vi "Test Panel Wavelength.vi"(8 "error in (no error)":errorcluster, 11 "VISA resource name":refnum<visa-resource-name>="COM4") -> (0 "error out":errorcluster, 3 "VISA resource name out":refnum<visa-resource-name>)   [LabVIEW 2017]
panel:
  out "Wavelength":dbl[unit]
  in  "Numeric":i32
  in  "stop":bool
  out "query output":string
  out "read buffer 3":string
  in  "wavelength":dbl[unit] min=0.0 max=1.99999e-05 step=1.0000000000000002e-10
  out "Boolean":bool
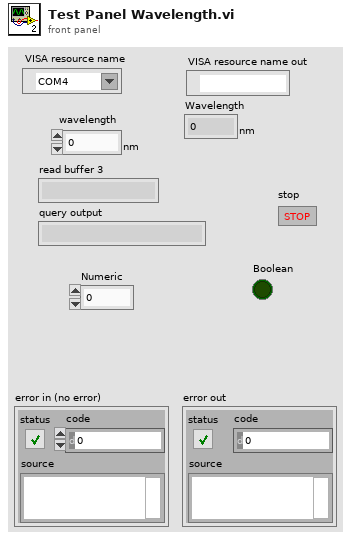
[diagram p1: front panel]
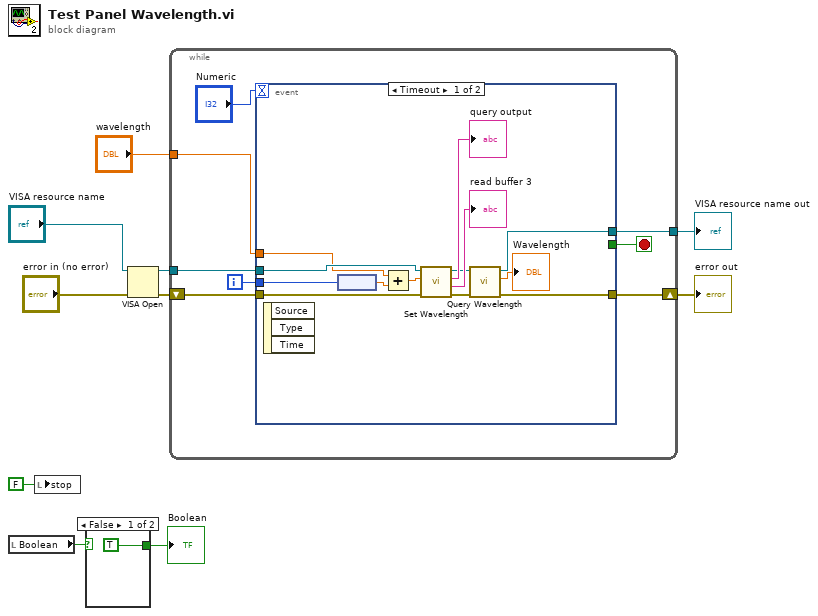
[diagram p0: block diagram]
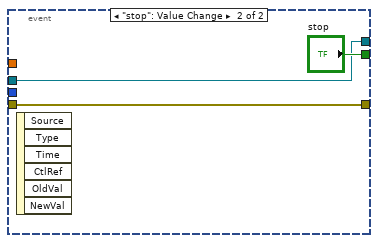
[diagram p2: hidden frame]
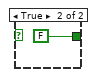
[diagram p3: hidden frame]
diagram:
  n1 = local read "Boolean"() -> (w8:bool)
  n2 = local write "stop"(FALSE ("stop")) -> ()
  n3 = case shown="False" w8 {
    tunnel: [TRUE FALSE] -> w7
    frame False {
    }
    frame True {
    }
  }
  "Boolean" <- w7
  n4 = VISA Open(error in (no error)="error in (no error)", VISA resource name="VISA resource name") -> (VISA resource name=w6:refnum<visa-resource-name>, error out=w5:errorcluster)  [unwired: 3 in]
  n5 = while {
    tunnel: w6 -> [w20]
    tunnel: [w17] -> w3
    tunnel: "wavelength" -> [w14]
    shift-right: [w18] -> w4
    shift-left: w5 -> [w19]
    i -> [w16]
    stop <- w15 stop-if-true
    n6 = event shown="[0] Timeout" {
      selector: _ -> [_ _]
      dyn-events: _ -> [_ _]
      timeout: "Numeric" -> [_ _]
      tunnel: w20 -> [w33 w35]
      tunnel: w19 -> [w32 w34]
      tunnel: [w22 w34] -> w18
      tunnel: [w23 w35] -> w17
      tunnel: w16 -> [w28 _]
      tunnel: [_ "stop"] -> w15
      tunnel: w14 -> [w26 _]
      event Timeout {
        n7 = event-data() -> ()  [unwired: 1 in, 3 out]
        n8 = node(w28) -> (w29:dbl[unit])
        n9 = Add(x=w26, y=w29) -> (x+y=w27:dbl[unit])
        n10 = call "Set Wavelength.vi"("error in (no error)"=w32, "wavelength"=w27, "VISA resource name"=w33) -> ("error out"=w25:errorcluster, "read buffer"=→"read buffer 3":string, "query output"=→"query output":string, "VISA resource name out"=w24:refnum<visa-resource-name>)  [unwired: 5 in]
        n11 = call "Query Wavelength.vi"("error in (no error)"=w25, "VISA resource name"=w24) -> ("error out"=w22:errorcluster, "Wavelength"=→"Wavelength":dbl[unit], "VISA resource name out"=w23:refnum<visa-resource-name>)  [unwired: 7 in]
      }
      event "stop": Value Change {
        n12 = event-data() -> ()  [unwired: 1 in, 6 out]
      }
    }
  }
  "error out" <- w4
  "VISA resource name out" <- w3
